vi "Gen_Trig_In.vi"(9 "Pulse width (clock pulses)":u8=200, 10 "Repeat Trigger":bool, 11 "Start":bool) -> (3 "Output":bool)   [LabVIEW 2020]
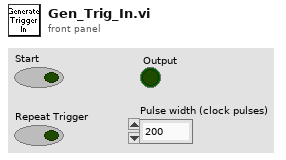
[diagram p1: front panel]
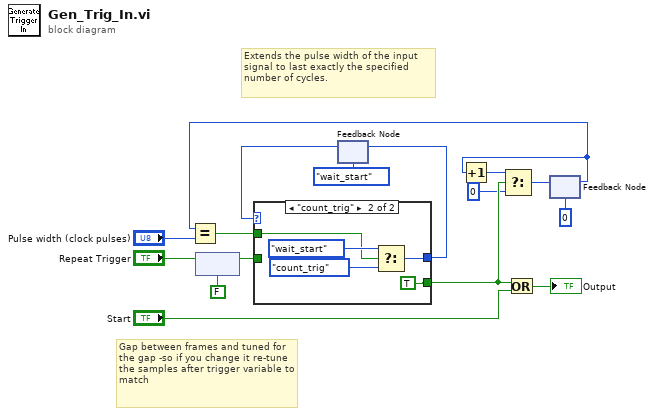
[diagram p0: block diagram]
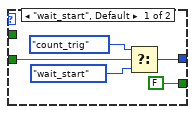
[diagram p2: hidden frame]
diagram:
  # "Gap between frames and tuned for the gap -so if you change it re-tune the samples after trigger variable to match"
  # "Extends the pulse width of the input signal to last exactly the specified number of cycles."
  n1 = feedback #1(FALSE ("repeat_trigger")) -> (w12:bool)
  n2 = feedback-in #1("Repeat Trigger") -> ()
  n3 = feedback #2(enum16{"wait_start", "count_trig"}."wait_start") -> (w4:enum16{"wait_start", "count_trig"})
  n4 = feedback #3(u8 0) -> (w2:u8)
  n5 = Equal?(x=w2, y="Pulse width (clock pulses)") -> (x = y?=w10:bool)
  n6 = case shown="\"count_trig\"" w4 {
    tunnel: w12 -> [w21 _]
    tunnel: [w19 w23] -> w3
    tunnel: [FALSE TRUE] -> w16
    tunnel: w10 -> [_ w22]
    frame "wait_start", Default {
      n7 = Select(t=enum16{"wait_start", "count_trig"}."count_trig", s=w21, f=enum16{"wait_start", "count_trig"}."wait_start") -> (s? t:f=w19:enum16{"wait_start", "count_trig"})
    }
    frame "count_trig" {
      n8 = Select(t=enum16{"wait_start", "count_trig"}."wait_start", s=w22, f=enum16{"wait_start", "count_trig"}."count_trig") -> (s? t:f=w23:enum16{"wait_start", "count_trig"})
    }
  }
  n9 = feedback-in #2(w3) -> ()
  n10 = Increment(x=w2) -> (x+1=w9:u8)
  n11 = Select(t=w9, s=w16, f=u8 0) -> (s? t:f=w7:u8)
  n12 = Or(x=w16, y="Start") -> (x .or. y?=→"Output":bool)
  n13 = feedback-in #3(w7) -> ()
